vi "AckermannPP.vi"(7 "Imaginary":dbl(knob)=-10.013861291935129 scale=0.0..-20.0 scale format="%#_4g", 8 "Real":dbl(knob)=-3.4076115316471642 scale=0.0..-22.0 scale format="%#_4g", 10 "State-Space Model":T4 {"Transport Delay" format="%.2f"; "D" format="%#.2g"; "C" format="%#.2g"; "B" format="%#.2g"; "A" format="%#.2g"; "properties"."Sampling Time" format="%#.6p"; "properties"."Output Delays" format="%.4f"; "properties"."Input Delays" format="%.4f"}) -> (0 "error out":errorcluster, 1 "Gain":dbl[](array[numeric]) format="%.3f", 2 "State Trajectory Graph":cluster{"time":dbl[], dbl[]}[](graph), 3 "Closed-Loop Step Response":cluster{"time":dbl[], dbl[]}[](graph), 4 "Actual Poles":cdb[](array[numeric])=[-4.9512521676495505+0.0i, -3.4076115316471447-10.013861291935113i, -3.4076115316471447+10.013861291935113i] format="%.2f", 5 "Time Response Parametric Data":T1={"Rise Time (s)"=[[0.0, 0.0], [0.0, 0.0]], "Peak Time (s)"=[[16.01539885840777, 17.159355919722614], [7.372167728473419, 117.70047097528251]], "Settling Time (s)"=[[0.0, 0.0], [0.0, 0.0]], "Overshoot (%)"=[[2.6933680524159342, 1.5395749934973058], [324.8704022191171, -0.0007732741527544107]], "Steady-State Gain"=[[0.0, 0.0], [0.0, 0.0]], "Peak Value"=[[0.0, 0.0], [0.0, 0.0]]}, 6 "Desired Poles":cdb[](array[numeric])=[-4.951252167649562+0.0i, -3.4076115316471642-10.013861291935129i, -3.4076115316471642+10.013861291935129i] format="%.2f")   [LabVIEW 2017]
uses:
  <vilib>/addons/Control Design/_Model Construction/Model Typedefs.llb/CD State Space Model (MIMO).ctl
  <vilib>/addons/Control Design/_Model Construction/Model Typedefs.llb/CD General Elements.ctl
  <vilib>/addons/Control Design/_Model Construction/Data Typedefs.llb/CD Plot Types Enum.ctl
  <vilib>/addons/Control Design/_Model Construction/Data Typedefs.llb/CD Parametric Time Response Data.ctl
  <vilib>/addons/Control Design/_Model Construction/Data Typedefs.llb/CD Time Info.ctl
  <vilib>/addons/Control Design/_State Feedback Control/State Feedback Control.llb/CD State Regulator.vi
  <vilib>/addons/Control Design/_Time Response Analysis/Time Response.llb/Time Response subVI/cd_Step Response (State-Space).vi
  <vilib>/addons/Control Design/_Time Response Analysis/Time Response.llb/Time Response subVI/cd_Parametric Time Response (SS).vi
  <vilib>/Analysis/NI_AALPro.lvlib
  <vilib>/addons/Control Design/_Model Construction/NI_LinSys_Data Typedefs.lvlib
  <vilib>/addons/Control Design/_Time Response Analysis/NI_CD_Time Response.lvlib
  <vilib>/addons/Control Design/_State Feedback Control/NI_CD_State Feedback Control.lvlib
  <vilib>/addons/Control Design/_Model Construction/NI_LinSys_Model Typedefs.lvlib
panel:
  out "Time Response Data":T3={"Time"=[], "Outputs Data"=[], "States Data"=[], "plot type"=enum."step"} {"States Data" format="%.2f"; "Outputs Data" format="%.2f"; "Time" format="%.2f"}
  out "Time Response":cluster{"time":dbl[], dbl[]}[](graph) caption="Time Response Graph"
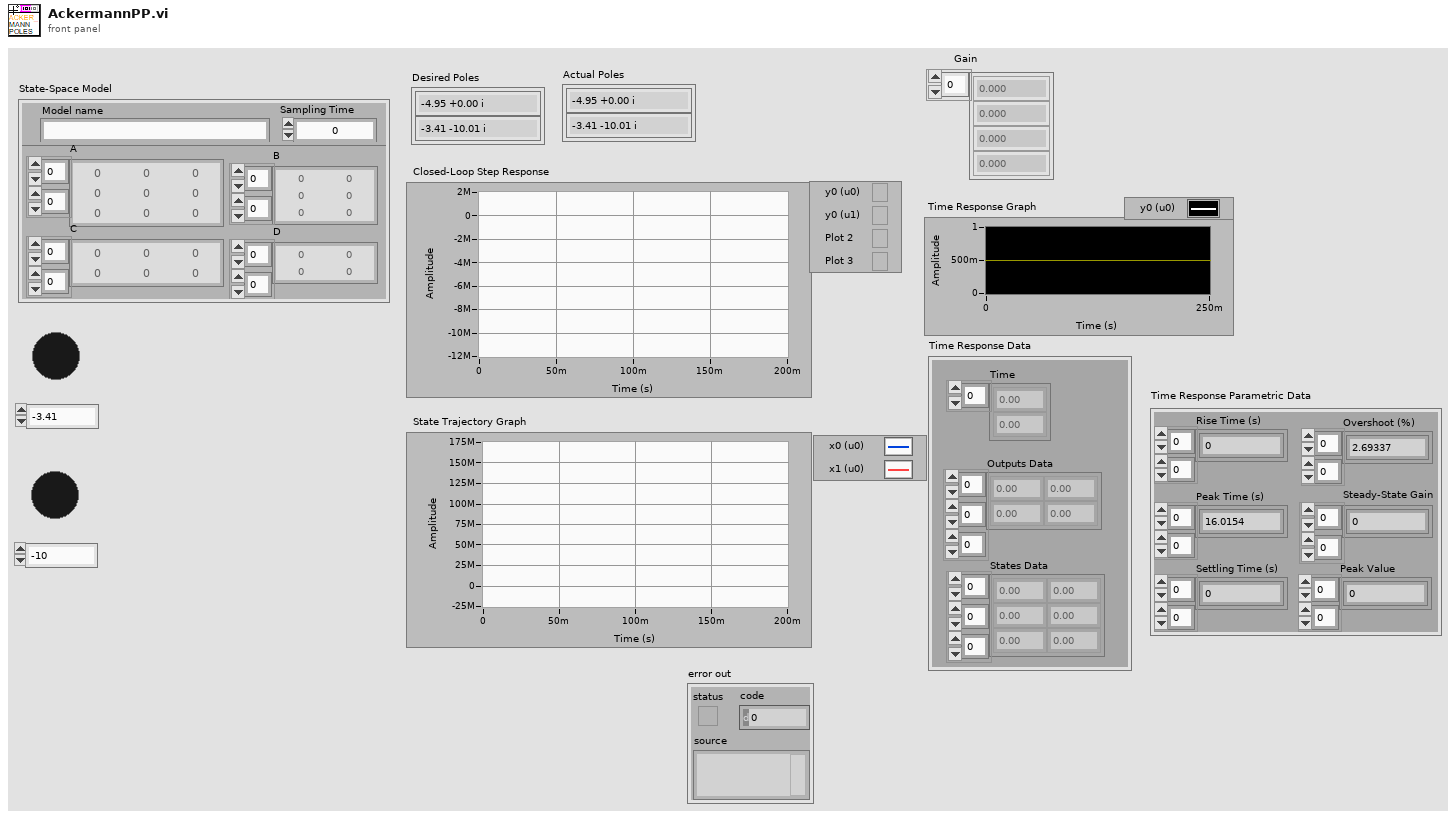
[diagram p1: front panel]
types:
  T1 = typedef "NI_LinSys_Data Typedefs.lvlib/CD Parametric Time Response Data.ctl" = cluster{"Rise Time (s)":dbl[][], "Peak Time (s)":dbl[][], "Settling Time (s)":dbl[][], "Overshoot (%)":dbl[][], "Steady-State Gain":dbl[][], "Peak Value":dbl[][]}
  T2 = typedef "NI_LinSys_Data Typedefs.lvlib/CD Plot Types Enum.ctl" = enum16{"bode-magnitude", "bode-phase", "nichols", "nyquist", "singular values", "step", "impulse", "initial", "simulation", "nyquist with separation"}
  T3 = cluster{"Time":dbl[], "Outputs Data":dbl[][][], "States Data":dbl[][][], "plot type":T2}
  T4 = typedef "NI_LinSys_Model Typedefs.lvlib/CD State Space Model (MIMO).ctl" = cluster{"properties":T5, "A":dbl[][], "B":dbl[][], "C":dbl[][], "D":dbl[][], "StateNames":string[], "Transport Delay":dbl[][]}
  T5 = typedef "NI_LinSys_Model Typedefs.lvlib/CD General Elements.ctl" = cluster{"Model name":string, "Input names":string[], "Output names":string[], "Input Delays":dbl[], "Output Delays":dbl[], "Sampling Time":dbl, "Notes":string}
  T6 = typedef "NI_LinSys_Data Typedefs.lvlib/CD Time Info.ctl" = cluster{"t0":dbl, "dt":dbl, "tf":dbl}
  T7 = enum16{"System Included", "System Included with Noise", "Standalone"}
  T8 = typedef "NI_Matrix.lvlib/RealMatrix.ctl" = dbl[][]
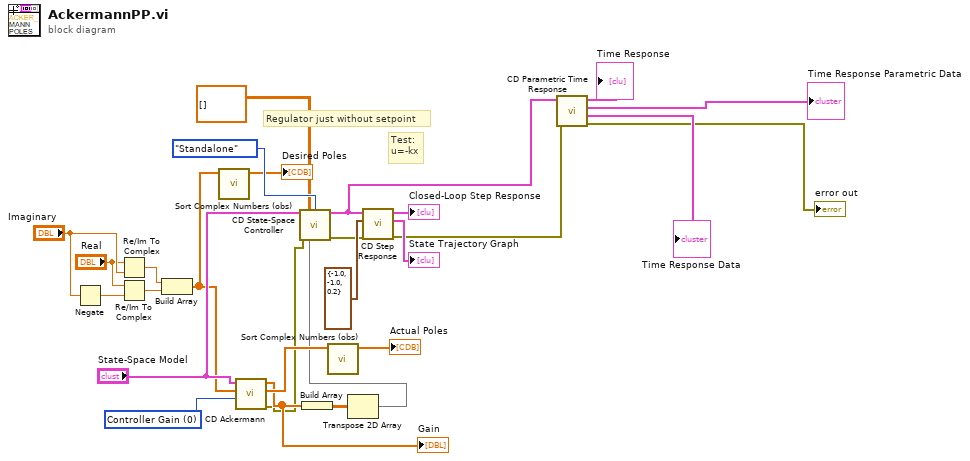
[diagram p0: block diagram]
diagram:
  w16 = u16 0 items=["Controller Gain", "Observer Gain (Predictive)", "Observer Gain (Current)"] ("Gain Type")
  # "Test:\nu=-kx"
  # "Regulator just without setpoint"
  n1 = Negate(x="Imaginary") -> (-x=w20:dbl)
  n2 = Re/Im To Complex(1:"Imaginary", 2:"Real") -> (0:w17:cdb)
  n3 = Re/Im To Complex(1:w20, 2:"Real") -> (0:w18:cdb)
  n4 = Build Array(w17, w18) -> (w14:cdb[])
  n5 = call <vilib>:"Sort Complex Numbers (obs).vi"("Complex Numbers"=w14) -> ("Sorted Complex Numbers"=→"Desired Poles":cdb[])  [unwired: 8 in, 2 out]
  n6 = call <vilib>:"CD Ackermann.vi"("Gain Type"=w16, "Poles"=w14, "State-Space Model"="State-Space Model") -> ("error out"=w4:errorcluster, "Actual Poles"=w13:cdb[], "Gain"=w11:dbl[])  [unwired: 6 in]
  "Gain" <- w11
  n7 = Build Array(w11) -> (w12:T8)
  n8 = call <vilib>:"Sort Complex Numbers (obs).vi"("Complex Numbers"=w13) -> ("Sorted Complex Numbers"=→"Actual Poles":cdb[])  [unwired: 8 in, 2 out]
  n9 = Transpose 2D Array(2D array=w12) -> (transposed array=w10:T8)
  n10 = call-poly <vilib>:"CD State-Space Controller.vi"("State-Space Model"="State-Space Model", "Estimator Gain (L)"=dbl[][] [], "Configuration"=T7."Standalone", "error in (no error)"=w4, "Controller Gain (K)"=w10) -> ("Controller Model"=w8:T4, "error out"=w3:errorcluster)  [unwired: 9 in]
  n11 = call-poly <vilib>:"CD Step Response.vi"("error in (no error)"=w3, "Time Range"=T6 {"t0"=-1.0, "dt"=-1.0, "tf"=0.2} ("Time Info"), "State-Space Model"=w8) -> ("error out"=w2:errorcluster, "State Trajectory Graph"=→"State Trajectory Graph":cluster{"time":dbl[], dbl[]}[], "Step Response Graph"=→"Closed-Loop Step Response":cluster{"time":dbl[], dbl[]}[])  [unwired: 5 in, 1 out]
  n12 = call-poly <vilib>:"CD Parametric Time Response.vi"("error in (no error)"=w2, "State-Space Model"=w8) -> ("error out"=→"error out":errorcluster, "Time Response Data"=→"Time Response Data":T3, "Time Response Parametric Data"=→"Time Response Parametric Data":T1, "Time Response"=→"Time Response":cluster{"time":dbl[], dbl[]}[])  [unwired: 6 in]
